vi "setNumberOfWheels.vi"(8 "error in (no error)":errorcluster, 10 "numberOfWheels":dbl, 11 "tricycle in":refnum<class "tricycle.lvclass">) -> (0 "error out":errorcluster, 3 "tricycle out":refnum<class "tricycle.lvclass">)   [LabVIEW 2011, in "tricycle.lvclass"]
uses:
  tricycle.lvclass
  genericVehicle.lvclass
  tricycle.lvclass/tricycle.ctl
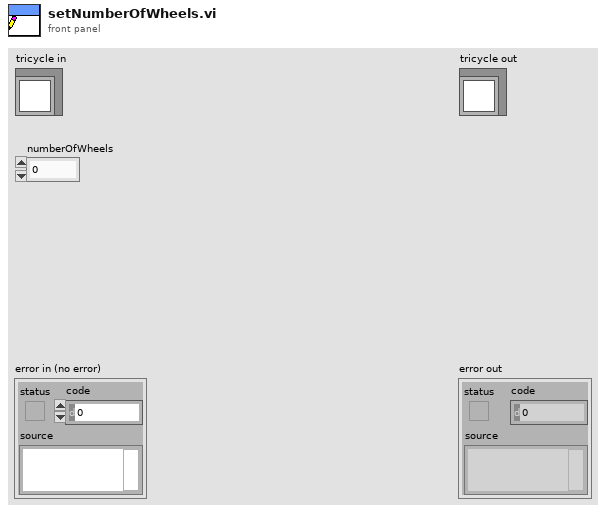
[diagram p1: front panel]
types:
  T1 = typedef "tricycle.ctl" = dbl
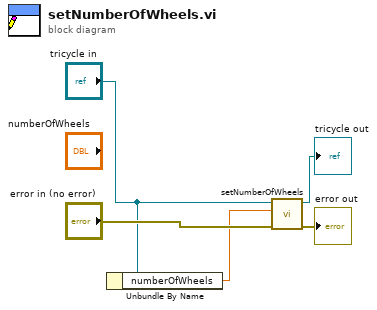
[diagram p0: block diagram]
diagram:
  n1 = Unbundle By Name("tricycle in") -> ("numberOfWheels"=w1:T1)
  n2 = call-parent "setNumberOfWheels.vi"("error in (no error)"="error in (no error)", "numberOfWheels"=w1, "genericVehicle in"="tricycle in") -> ("error out"=→"error out":errorcluster, "genericVehicle out"=→"tricycle out":refnum<class "tricycle.lvclass">)  [unwired: 7 in]
